vi "Esercizio lezione 1-2 random.vi"(1 "Offset":dbl, 2 "Input":dbl caption="Numeric" format="%#.1g") -> (0 "Output":dbl)   [LabVIEW 2012]
panel:
  # "ESERCIZIO 1-2"
  # "- nome del VI ran (anche in icona)\n- calcolare prodotto di un numero intero (input) per il valore fornito da un generatore di numeri casuali,\nsommare al risultato il valore della variabile (offset) e inviare il numero risultante alla variabile (output)\n- indicatori e controlli devono essere collegati al connettore"
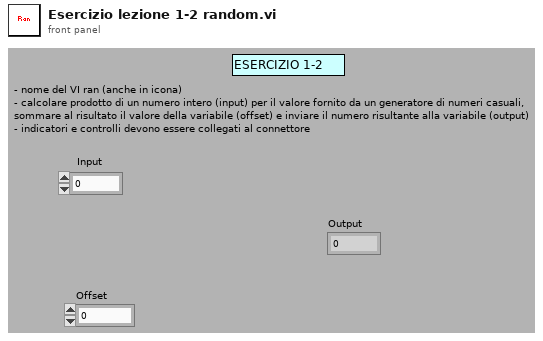
[diagram p1: front panel]
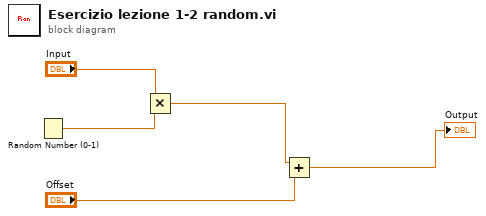
[diagram p0: block diagram]
diagram:
  n1 = Random Number (0-1)() -> (number: 0 to 1=w5:dbl)
  n2 = Multiply(x="Input", y=w5) -> (x*y=w4:dbl)
  n3 = Add(x=w4, y="Offset") -> (x+y=→"Output":dbl)
